vi "Check Server Validity.vi"(8 "error in (no error)":errorcluster, 11 "Server URL":refnum<k21>) -> (0 "error out":errorcluster, 1 "Valid?":bool, 3 "dup Server URL":refnum<k21>)   [LabVIEW 2024]
doc: "Checks whether a server is valid."
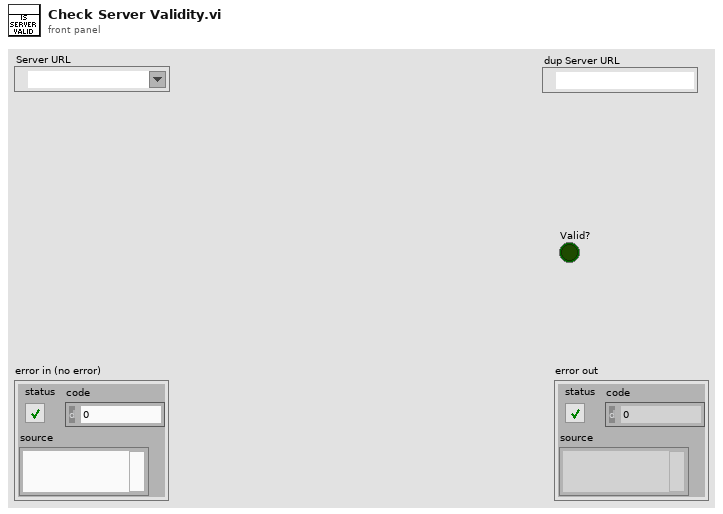
[diagram p1: front panel]
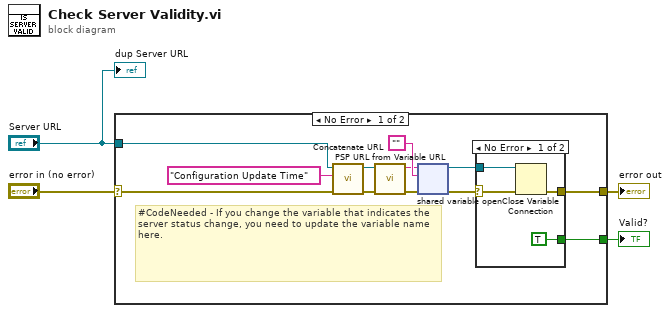
[diagram p0: block diagram]
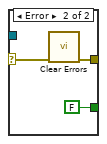
[diagram p2: hidden frame]
diagram:
  n1 = case shown="No Error" "error in (no error)" {
    selector: "error in (no error)" -> [w16 w24]
    tunnel: [w5 w24] -> w3
    tunnel: "Server URL" -> [w15 _]
    tunnel: [w14 _] -> w1
    frame No Error {
      # "#CodeNeeded - If you change the variable that indicates the server status change, you need to update the variable name here."
      n2 = call "Concatenate URL.vi"("error in (no error)"=w16, "Child Name"="Configuration Update Time", "Parent URL"=w15) -> ("error out"=w13:errorcluster, "Child URL"=w9:refnum<k21>)  [unwired: 7 in]
      n3 = call "PSP URL from Variable URL.vi"("error in (no error)"=w13, "Shared Variable URL"=w9) -> ("error out"=w12:errorcluster, "PSP URL"=w10:string)  [unwired: 8 in]
      n4 = shared-variable-open(w10, w12, "" ("y")) -> (w6:refnum<k21>, w7:errorcluster)  [unwired: 1 in]
      n5 = case shown="No Error" w7 {
        selector: w7 -> [w19 w22]
        tunnel: [TRUE ("Valid?") FALSE ("Valid?")] -> w14
        tunnel: w6 -> [w18 _]
        tunnel: [w17 w21] -> w5
        frame No Error {
          n6 = Close Variable Connection(8:w19, 11:w18) -> (0:w17:errorcluster)
        }
        frame Error {
          n7 = call <vilib>:"Clear Errors.vi"("error in (no error)"=w22) -> ("error out"=w21:errorcluster)  [unwired: 5 in, 1 out]
        }
      }
    }
    frame Error {
    }
  }
  "error out" <- w3
  "Valid?" <- w1
  "dup Server URL" <- "Server URL"
